vi "Senal_Triangular_Ciclo_For.vi"() -> ()   [LabVIEW 2016]
panel:
  in  "Offset":dbl(knob) scale=0.0..10.0
  in  "Frecuencia":dbl(knob) scale=0.0..10.0
  in  "Muestras":i32(slide) scale=10.0..1000.0
  in  "Amplitud":dbl(knob) scale=-10.0..10.0
  out "Waveform Graph":dbl[](graph)
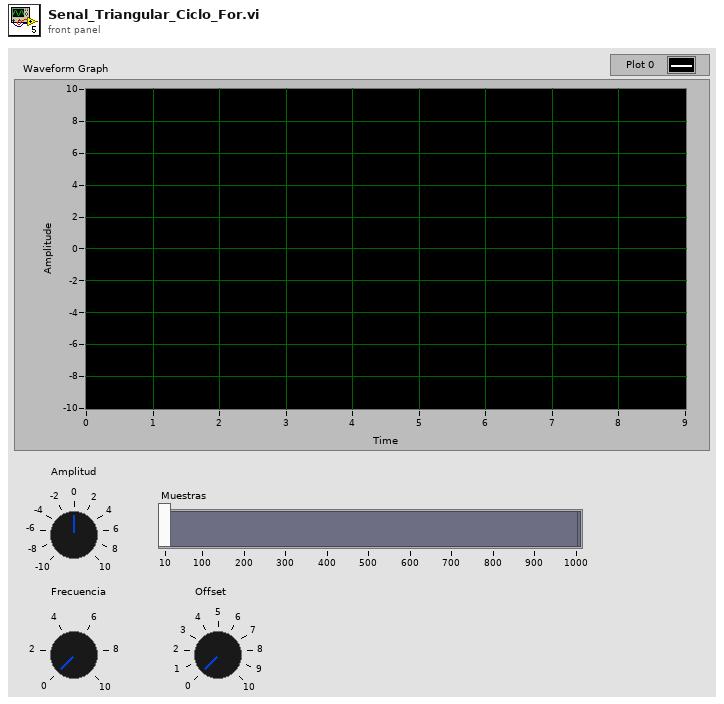
[diagram p1: front panel]
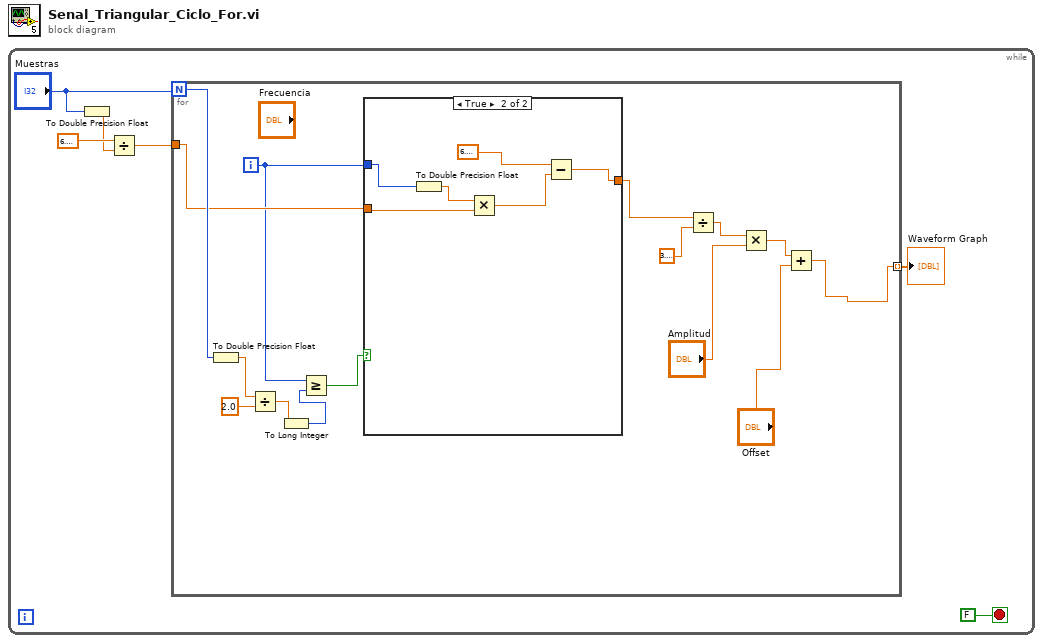
[diagram p0: block diagram]
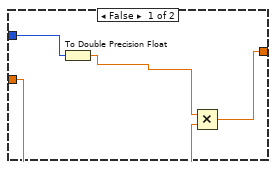
[diagram p2: hidden frame]
diagram:
  n1 = while {
    stop <- FALSE stop-if-true
    n2 = To Double Precision Float(number="Muestras") -> (double precision float=w2:dbl)
    n3 = Divide(x=6.283185307179586, y=w2) -> (x/y=w1:dbl)
    n4 = for {
      N: "Muestras" -> [w16]
      tunnel: [w9] -> w5 mode=indexing
      tunnel: w1 -> [w15]
      i -> [w7]
      n5 = To Double Precision Float(number=w16) -> (double precision float=w17:dbl)
      n6 = Divide(x=w17, y=2.0) -> (x/y=w20:dbl)
      n7 = To Long Integer(number=w20) -> (32bit integer=w19:i32)
      n8 = Greater Or Equal?(x=w7, y=w19) -> (x >= y?=w21:bool)
      n9 = case shown="True" w21 {
        tunnel: w15 -> [w22 w30]
        tunnel: w7 -> [w25 w29]
        tunnel: [w24 w27] -> w8
        frame False {
          n10 = To Double Precision Float(number=w25) -> (double precision float=w23:dbl)
          n11 = Multiply(x=w23, y=w22) -> (x*y=w24:dbl)
        }
        frame True {
          n12 = To Double Precision Float(number=w29) -> (double precision float=w31:dbl)
          n13 = Multiply(x=w31, y=w30) -> (x*y=w26:dbl)
          n14 = Subtract(x=6.283185307179586, y=w26) -> (x-y=w27:dbl)
        }
      }
      n15 = Divide(x=w8, y=3.141592653589793) -> (x/y=w13:dbl)
      n16 = Multiply(x=w13, y="Amplitud") -> (x*y=w11:dbl)
      n17 = Add(x=w11, y="Offset") -> (x+y=w9:dbl)
    }
    "Waveform Graph" <- w5
  }
